vi "Converter_add_to_sum_array.vi"(9 "Sum array in":T1, 10 "Data in (11vals)":dbl[](array[numeric]), 11 "Data from unit":i32) -> (1 "Sum array":T1)   [LabVIEW 2013]
doc: "this VI receives data from unit and sums array. \n*finds if unit is in array\n *if yes, adds values to currently presents\n , increments index 0 - number of additions\n *if no, creates new column for the unit and orders the array to have unit numbers in order"
uses:
  Sum_array_for_avg_baseline.ctl
panel:
  out "Boolean":bool
  out "Numeric":i32
  out "index of element":i32
  # "this VI receives data from unit and sums array. \n*finds if unit is in array\n  *if yes, adds values to currently presents\n             , increments index 0 - number of additions\n  *if no, creates new column for the unit and orders the array to have unit numbers in order"
  # "index0 - number of additions"
  # "index1 - unit number"
  # "A1.0"
  # "A1.1"
  # "index13 A3.3"
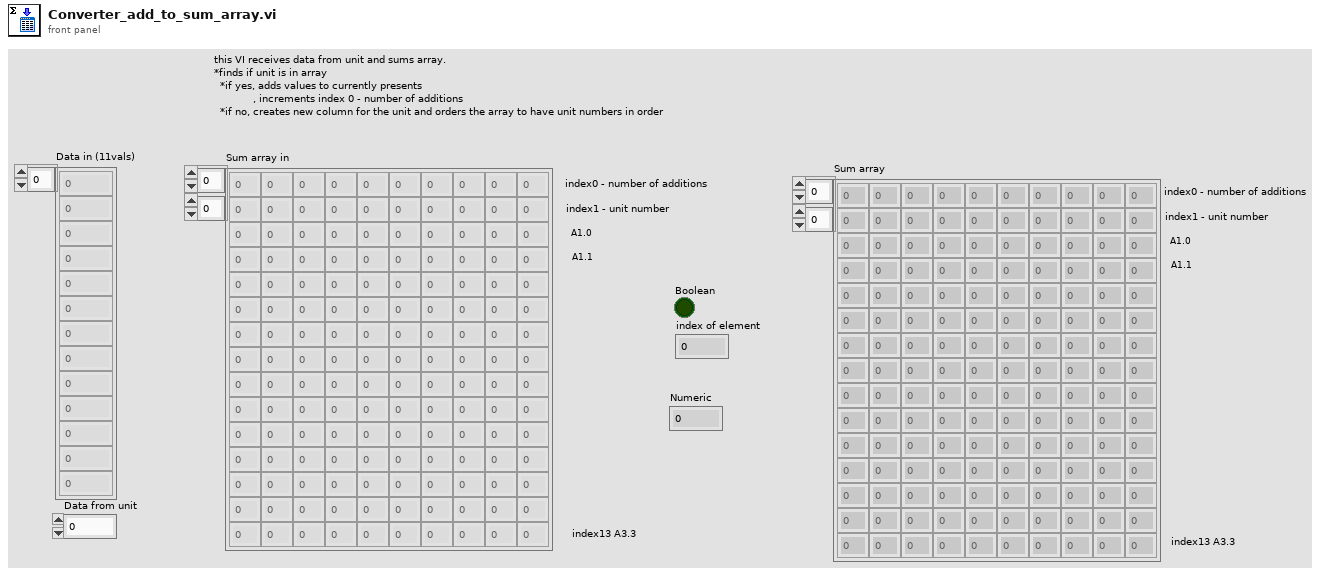
[diagram p1: front panel]
types:
  T1 = typedef "Sum_array_for_avg_baseline.ctl" = dbl[][]
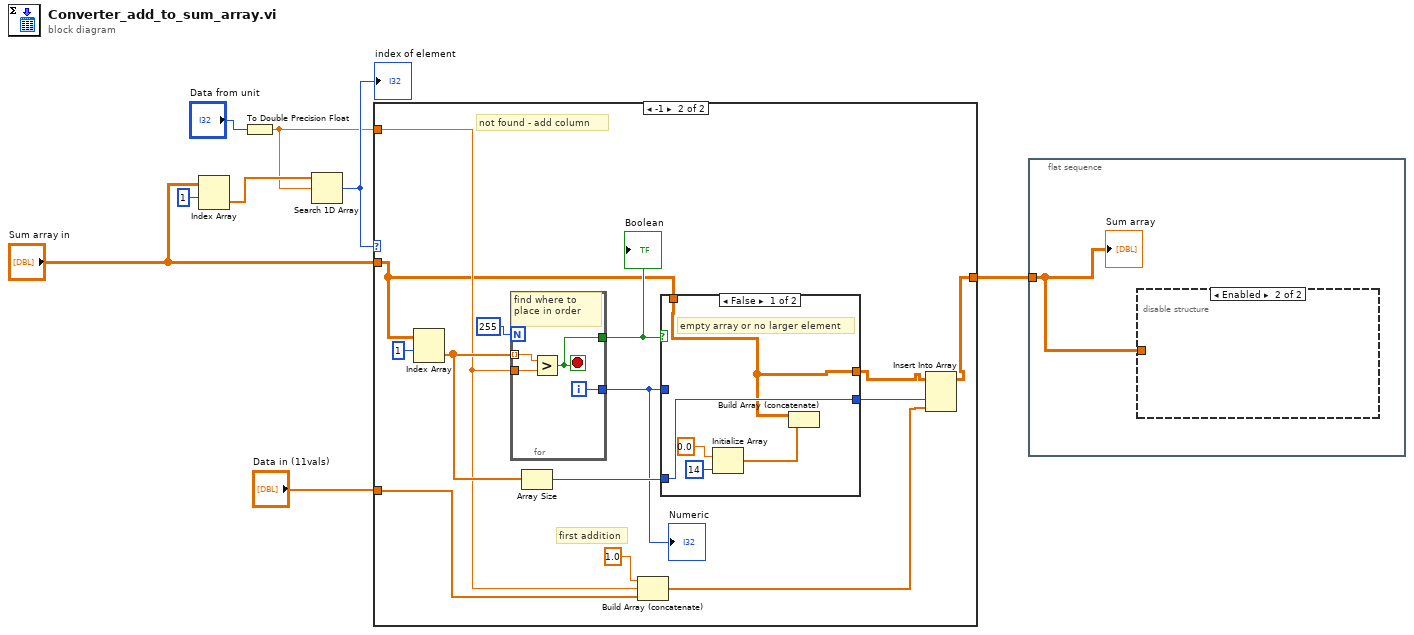
[diagram p0: block diagram]
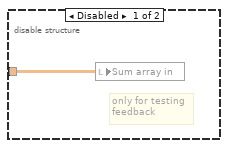
[diagram p2: hidden frame]
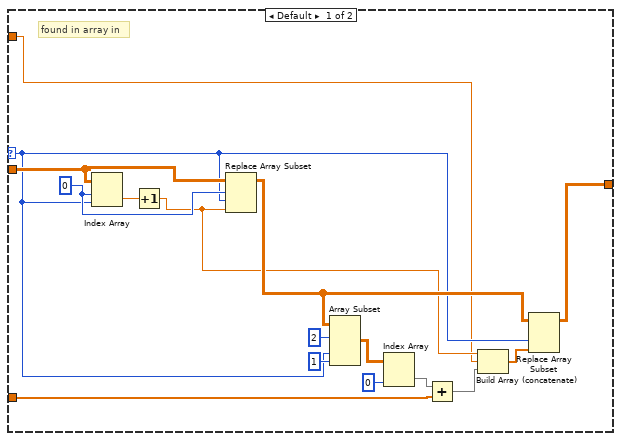
[diagram p3: hidden frame]
diagram:
  n1 = Index Array(array="Sum array in", index (row)=1) -> (element=w7:dbl[])  [unwired: 1 in]
  n2 = To Double Precision Float(number="Data from unit") -> (double precision float=w1:dbl)
  n3 = Search 1D Array(1D array=w7, element=w1) -> (index of element=w5:i32)  [unwired: 1 in]
  "index of element" <- w5
  n4 = case shown="-1" w5 {
    selector: w5 -> [w13 _]
    tunnel: "Sum array in" -> [w16 w30]
    tunnel: [w14 w28] -> w3
    tunnel: "Data in (11vals)" -> [w17 w31]
    tunnel: w1 -> [w9 w32]
    frame Default {
      w23 = 0 ("index (row)")
      # "found in array in"
      n5 = Index Array(array=w16, index (row)=w23, index (col)=w13) -> (element=w24:dbl)
      n6 = Increment(x=w24) -> (x+1=w10:dbl)
      n7 = Replace Array Subset(array=w16, new element=w10, index (row)=w23, index (col)=w13) -> (w15:T1)
      n8 = Array Subset(array=w15, index (row)=2 ("index"), index (col)=w13, length (col)=1 ("length")) -> (w20:T1)  [unwired: 1 in]
      n9 = Index Array(array=w20, index (col)=0 ("disabled index (col)")) -> (element=w18:dbl[])  [unwired: 1 in]
      n10 = Add(x=w18, y=w17) -> (x+y=w12:dbl[])
      n11 = Build Array (concatenate)(w10, w9, w12) -> (w11:dbl[])
      n12 = Replace Array Subset(array=w15, new element=w11, index (col)=w13) -> (w14:T1)  [unwired: 1 in]
    }
    frame -1 {
      # "first addition"
      # "not found - add column"
      n13 = Index Array(array=w30, index (row)=1) -> (element=w35:dbl[])  [unwired: 1 in]
      n14 = for {
        N: 255 -> [_]
        tunnel: w35 -> [w49] mode=indexing
        tunnel: w32 -> [w48]
        tunnel: [w47] -> w25
        tunnel: [w46] -> w36
        i -> [w47]
        stop <- w46 stop-if-true
        # "find where to place in order"
        n15 = Greater?(x=w49, y=w48) -> (0:w46:bool)
      }
      "Numeric" <- w25
      "Boolean" <- w36
      n16 = Array Size(array=w35) -> (size(s)=w34:i32)
      n17 = Build Array (concatenate)(1.0 ("element"), w32, w31) -> (w26:dbl[])
      n18 = case shown="False" w36 {
        tunnel: w25 -> [_ w45]
        tunnel: w34 -> [w43 _]
        tunnel: [w43 w45] -> w27
        tunnel: w30 -> [w39 w44]
        tunnel: [w39 w44] -> w29
        frame False {
          # "empty array or no larger element"
          n19 = Initialize Array(0.0 ("element"), 14 ("dimension size")) -> (w40:dbl[])
          n20 = Build Array (concatenate)(w39, w40) -> ()  [unwired: 1 out]
        }
        frame True {
          # "index known where to put"
        }
      }
      n21 = Insert Into Array(array=w29, index (col)=w27, new element=w26) -> (w28:T1)  [unwired: 1 in]
    }
  }
  n22 = flat-sequence {
    tunnel: w3 -> [w50]
    frame #0 {
      n23 = disable-structure shown="Enabled" {
        disable-tunnel: w50 -> [w51 _]
        frame Disabled {
          # "only for testing\nfeedback"
          n24 = local write "Sum array in"(w51) -> ()
        }
        frame Enabled {
        }
      }
      "Sum array" <- w50
    }
  }
